vi "tool list.vi"(8 "error in":errorcluster, 10 "server id in":i32, 11 "message json":string) -> (0 "error out":errorcluster, 3 "response":string)   [LabVIEW 2025, in "MCP Server.lvlib"]
uses:
  MCP Server.lvlib
  8dc8bba5-80dd-4b6d-92c4-f894be10601f.vi
  501006b8-601a-4e2b-b374-4fa6edd3fcfa.vi
  67376cc4-96dd-428d-b57d-13d5d9c2dcda.vi
  457f7257-2385-409f-8748-2a948732079c.vi
  072bd452-694b-4df1-bacb-9596dea07f88.vi
  <vilib>/JDP Science/JSONtext/Variant to JSON Text.vi
  <vilib>/JDP Science/JSONtext/Set Multiple Object Items.vi
  <vilib>/JDP Science/JSONtext/Get all Object Items.vi
  <vilib>/JDP Science/JSONtext/support/Format JSON Array Text.vi
  <vilib>/JDP Science/JSONtext/support/Format JSON Object.vi
  <vilib>/JDP Science/JSONtext/LVClass Serializer/JSONtext LVClass Serializer.lvclass
  <vilib>/JDP Science/JSONtext/JSONtext.lvlib
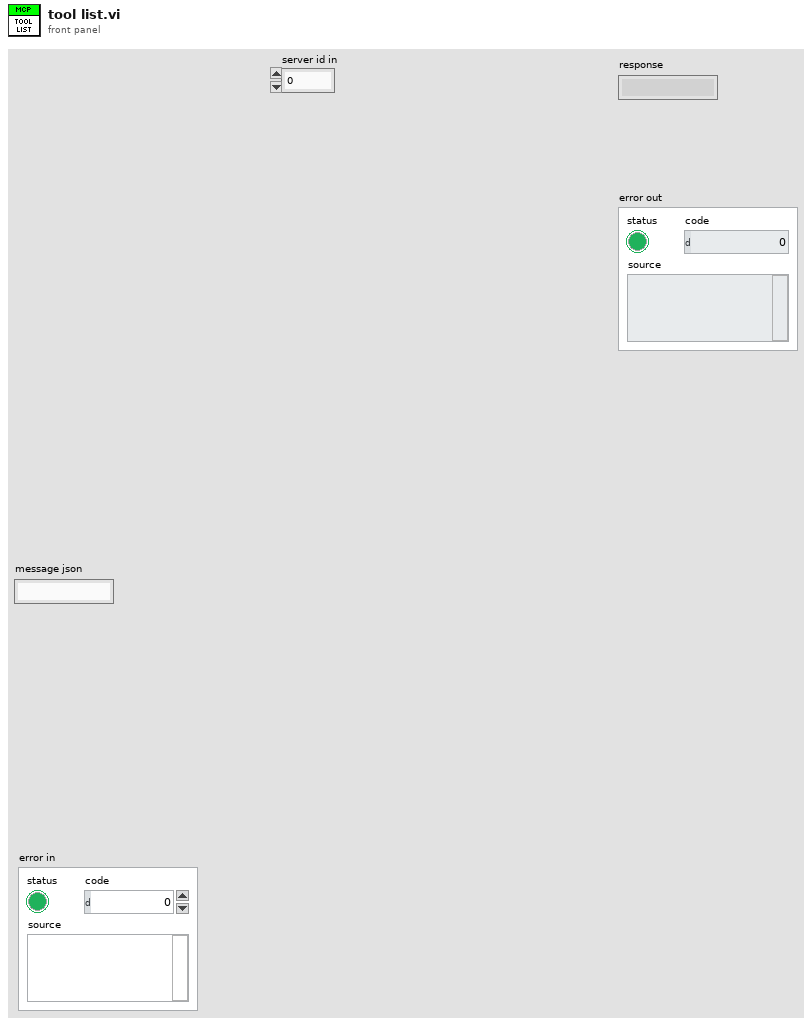
[diagram p1: front panel]
types:
  T1 = typedef "MCP Server.lvlib/Tool Data.ctl" = cluster{"Name":string, "Description":string, "Ignored":string[], "inputs":T2[], "outputs":T3[], "VI Refnum":refnum<vi>}
  T2 = typedef "MCP Server.lvlib/Input Parameter.ctl" = cluster{"name":string, "type":string, "description":string, "required":bool, "raw name":string}
  T3 = typedef "MCP Server.lvlib/Output Parameter.ctl" = cluster{"name":string, "description":string, "type":string, "raw name":string}
  T4 = cluster{"name":string, "title":string, "description":string}
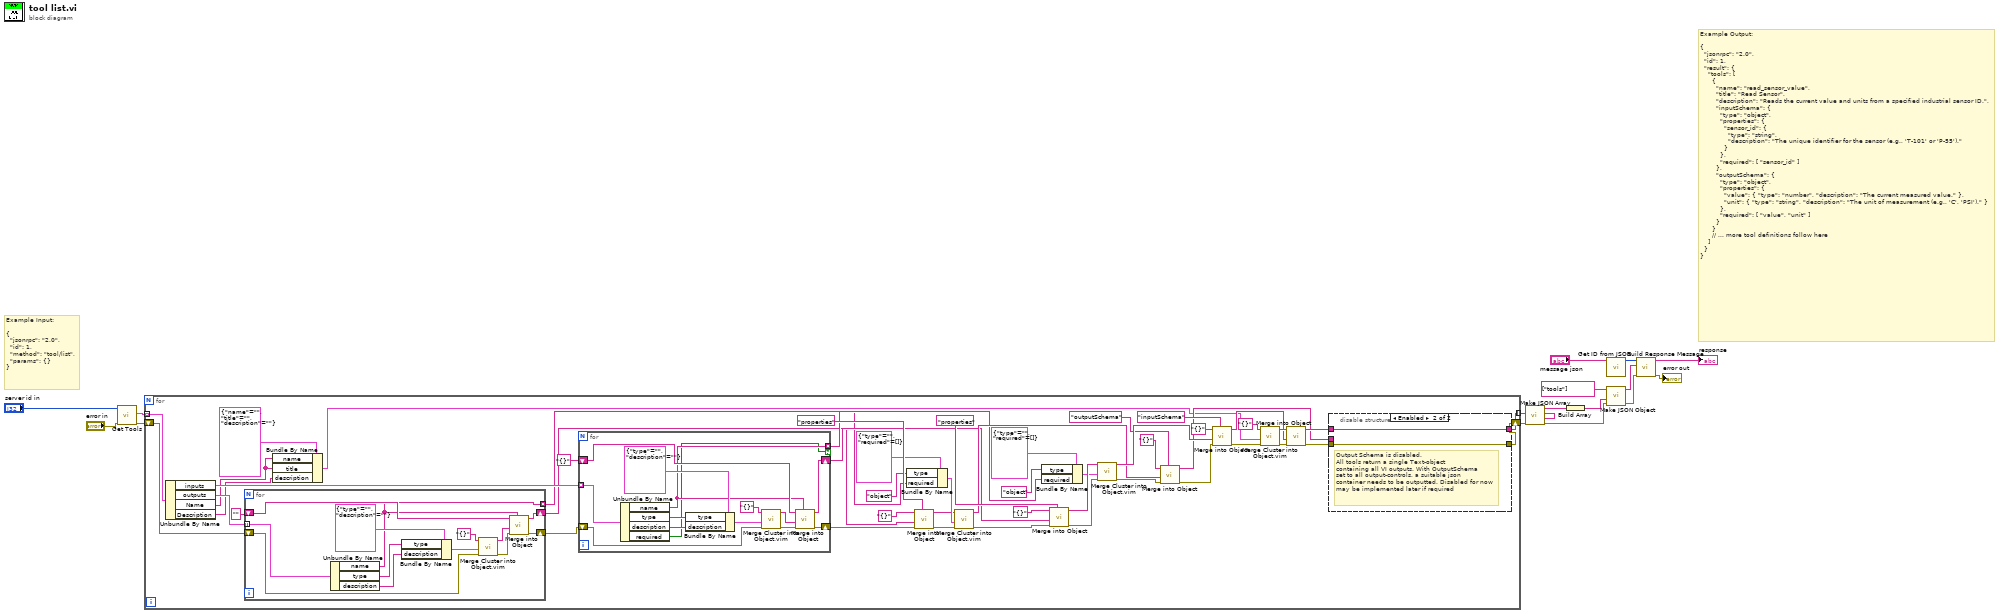
[diagram p0: block diagram]
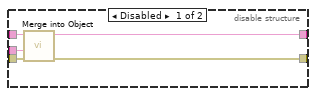
[diagram p2: hidden frame]
diagram:
  # "Example Output:\n\n{\n  \"jsonrpc\": \"2.0\",\n  \"id\": 1,\n  \"result\": {\n    \"tools\": [\n      {\n        \"name\": \"read_sensor_value\",\n        \"title\": \"Read Sensor\",\n        \"description\": \"Reads the current value and units from a specified industrial sensor ID.\",\n        \"inputSchema\": {\n          \"type\": \"object\",\n          \"properties\": {\n            \"sensor_id\": {\n              \"type\": \"string\",\n              \"description\": \"The unique identifier for the sensor (e.g., 'T-101' or 'P-55').\"\n            }\n          },\n          \"required\": [ \"sensor_id\" ]\n        },\n        \"outputSchema\": {\n          \"type\": \"object\",\n          \"properties\": {\n            \"value\": { \"type\": \"number\", \"description\": \"The current measured value.\" },\n            \"unit\": { \"type\": \"string\", \"description\": \"The unit of measurement (e.g., 'C', 'PSI').\" }\n          },\n          \"required\": [ \"value\", \"unit\" ]\n        }\n      }\n      // ... more tool definitions follow here\n    ]\n  }\n}"
  # "Example Input:\n\n{\n  \"jsonrpc\": \"2.0\",\n  \"id\": 1,\n  \"method\": \"tool/list\",\n  \"params\": {}\n}"
  n1 = call "Get Tools.vi"("error in (no error)"="error in", "server id in"="server id in") -> ("error out"=w13:errorcluster, "Tools"=w12:T1[])  [unwired: 7 in, 1 out]
  n2 = for {
    tunnel: w12 -> [w65] mode=indexing
    shift-right: [w27] -> w7
    shift-left: w13 -> [w28]
    tunnel: [w39] -> w11 mode=indexing
    n3 = Unbundle By Name(w65) -> ("inputs"=w37:T2[], "outputs"=w33:T3[], "Name"=w31:string, "Description"=w32:string)
    n4 = for {
      tunnel: w33 -> [w80] mode=indexing
      shift-right: [w85] -> w34
      shift-left: "" ("<JSON>") -> [w84]
      tunnel: [w76] -> w30 mode=indexing
      shift-right: [w74] -> w29
      shift-left: w28 -> [w73]
      n5 = Unbundle By Name(w80) -> ("name"=w76:string, "type"=w79:string, "description"=w78:string)
      n6 = Bundle By Name(cluster=cluster{"type":string, "description":string} {"type"="", "description"=""}, "type"=w79, "description"=w78) -> (w83:cluster{"type":string, "description":string})
      n7 = call "Merge Cluster into Object.vim"("error in (no error)"=w73, "Any Cluster"=w83, "JSON"="{}") -> ("error out"=w75:errorcluster, "<JSON>"=w77:string)  [unwired: 6 in]
      n8 = call <vilib>:"Merge into Object.vi"("$Path or Item Name"=w76, "error in (no error)"=w75, "JSON Object to Merge"=w77, "JSON"=w84) -> ("error out"=w74:errorcluster, "<JSON>"=w85:string)  [unwired: 5 in]
    }
    n9 = Bundle By Name(cluster=T4 {"name"="", "title"="", "description"=""}, "name"=w31, "title"=w31, "description"=w32) -> (w40:T4)
    n10 = for {
      tunnel: w37 -> [w94] mode=indexing
      shift-right: [w99] -> w35
      shift-left: "{}" ("<JSON>") -> [w98]
      tunnel: [w90] -> w36 mode=indexing if=w89
      shift-right: [w87] -> w18
      shift-left: w29 -> [w86]
      n11 = Unbundle By Name(w94) -> ("name"=w90:string, "type"=w93:string, "description"=w92:string, "required"=w89:bool)
      n12 = Bundle By Name(cluster=cluster{"type":string, "description":string} {"type"="", "description"=""}, "type"=w93, "description"=w92) -> (w97:cluster{"type":string, "description":string})
      n13 = call "Merge Cluster into Object.vim"("error in (no error)"=w86, "Any Cluster"=w97, "JSON"="{}") -> ("error out"=w88:errorcluster, "<JSON>"=w91:string)  [unwired: 6 in]
      n14 = call <vilib>:"Merge into Object.vi"("$Path or Item Name"=w90, "error in (no error)"=w88, "JSON Object to Merge"=w91, "JSON"=w98) -> ("error out"=w87:errorcluster, "<JSON>"=w99:string)  [unwired: 5 in]
    }
    n15 = Bundle By Name(cluster=cluster{"type":string, "required":string[]} {"type"="", "required"=[]}, "type"="object", "required"=w30) -> (w51:cluster{"type":string, "required":string[]})
    n16 = call <vilib>:"Merge into Object.vi"("$Path or Item Name"="properties", "error in (no error)"=w18, "JSON Object to Merge"=w34, "JSON"="{}") -> ("error out"=w19:errorcluster, "<JSON>"=w50:string)  [unwired: 5 in]
    n17 = call "Merge Cluster into Object.vim"("error in (no error)"=w19, "Any Cluster"=w51, "JSON"=w50) -> ("error out"=w20:errorcluster, "<JSON>"=w47:string)  [unwired: 6 in]
    n18 = Bundle By Name(cluster=cluster{"type":string, "required":string[]} {"type"="", "required"=[]}, "type"="object", "required"=w36) -> (w57:cluster{"type":string, "required":string[]})
    n19 = call <vilib>:"Merge into Object.vi"("$Path or Item Name"="properties", "error in (no error)"=w20, "JSON Object to Merge"=w35, "JSON"="{}") -> ("error out"=w21:errorcluster, "<JSON>"=w60:string)  [unwired: 5 in]
    n20 = call "Merge Cluster into Object.vim"("error in (no error)"=w21, "Any Cluster"=w57, "JSON"=w60) -> ("error out"=w22:errorcluster, "<JSON>"=w55:string)  [unwired: 6 in]
    n21 = call <vilib>:"Merge into Object.vi"("$Path or Item Name"="outputSchema", "error in (no error)"=w22, "JSON Object to Merge"=w47, "JSON"="{}") -> ("error out"=w23:errorcluster, "<JSON>"=w43:string)  [unwired: 5 in]
    n22 = call <vilib>:"Merge into Object.vi"("$Path or Item Name"="inputSchema", "error in (no error)"=w23, "JSON Object to Merge"=w55, "JSON"="{}") -> ("error out"=w24:errorcluster, "<JSON>"=w44:string)  [unwired: 5 in]
    n23 = call "Merge Cluster into Object.vim"("error in (no error)"=w24, "Any Cluster"=w40, "JSON"="{}") -> ("error out"=w25:errorcluster, "<JSON>"=w46:string)  [unwired: 6 in]
    n24 = call <vilib>:"Merge into Object.vi"("error in (no error)"=w25, "JSON Object to Merge"=w44, "JSON"=w46) -> ("error out"=w26:errorcluster, "<JSON>"=w45:string)  [unwired: 6 in]
    n25 = disable-structure shown="Enabled" {
      disable-tunnel: w45 -> [w70 w71]
      disable-tunnel: w43 -> [w69 _]
      disable-tunnel: [w68 w71] -> w39
      disable-tunnel: [w67 w72] -> w27
      disable-tunnel: w26 -> [w66 w72]
      frame Disabled {
        n26 = call <vilib>:"Merge into Object.vi"("error in (no error)"=w66, "JSON Object to Merge"=w69, "JSON"=w70) -> ("error out"=w67:errorcluster, "<JSON>"=w68:string)  [unwired: 6 in]
      }
      frame Enabled {
        # "Output Schema is disabled.\nAll tools return a single Text-object\ncontaining all VI outputs. With OutputSchema\nset to all output-controls, a suitable json \ncontainer needs to be outputted. Disabled for now\nmay be implemented later if required"
      }
    }
  }
  n27 = call <vilib>:"Make JSON Array.vi"("error in (no error)"=w7, "JSON Elements"=w11) -> ("error out"=w6:errorcluster, "<JSON>"=w9:string)  [unwired: 8 in]
  n28 = Build Array(w9) -> (w8:string[])
  n29 = call "Get ID from JSON.vi"("message json"="message json") -> ("Data out"=w2:i32)  [unwired: 10 in]
  n30 = call <vilib>:"Make JSON Object.vi"("error in (no error)"=w6, "JSON Items"=w8, "Item Names"=string[] ["tools"]) -> ("error out"=w5:errorcluster, "<JSON>"=w1:string)  [unwired: 7 in]
  n31 = call "Build Response Message.vi"("error in (no error)"=w5, "Result content"=w1, "message id in"=w2) -> ("error out"=→"error out":errorcluster, "MCP message out"=→"response":string)  [unwired: 7 in]
